vi "Add Prefix.vi"(2 "If Empty":string="Cluster", 7 "Name in":string, 13 "Prefix":string) -> (8 "Name out":string)   [LabVIEW 2017, in "TreeLUT.lvclass"]
uses:
  TreeLUT.lvclass
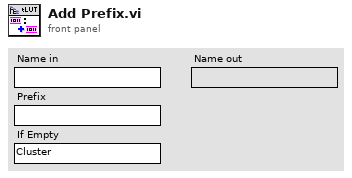
[diagram p1: front panel]
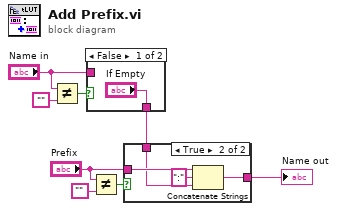
[diagram p0: block diagram]
diagram:
  n1 = Not Equal?(x="Name in", y="") -> (x != y?=w3:bool)
  n2 = case shown="False" w3 {
    tunnel: "Name in" -> [_ w10]
    tunnel: ["If Empty" w10] -> w1
    frame False {
    }
    frame True {
    }
  }
  n3 = Not Equal?(x="Prefix", y="") -> (x != y?=w7:bool)
  n4 = case shown="True" w7 {
    tunnel: w1 -> [w11 w14]
    tunnel: [w11 w12] -> w5
    tunnel: "Prefix" -> [_ w15]
    frame False {
    }
    frame True {
      n5 = Concatenate Strings(w15, ":" ("string"), w14) -> (w12:string)
    }
  }
  "Name out" <- w5
